vi "tm_readmetadata.vi"(5 "Index":i32, 7 "Type":i32(ring) items=["FILE"=0, "FRAME"=2], 8 "error in (no error)":errorcluster, 11 "File Handle":u32) -> (0 "error out":errorcluster, 2 "Metadata":string, 3 "File Handle":u32)   [LabVIEW 2011]
uses:
  tmcamcon.dll
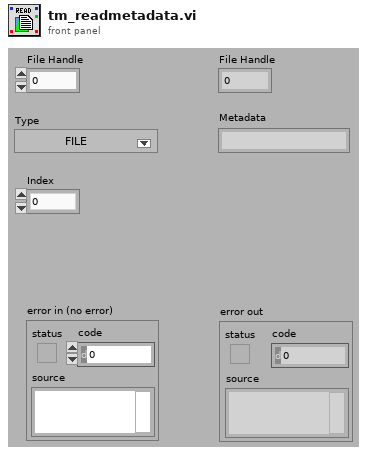
[diagram p1: front panel]
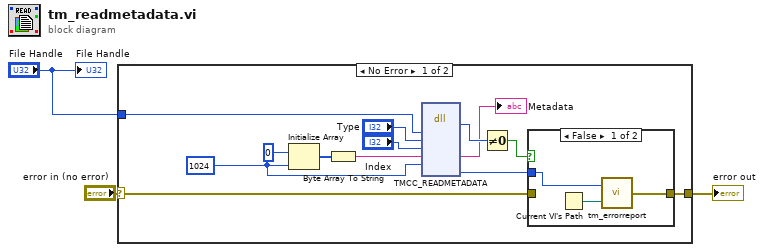
[diagram p0: block diagram]
diagram:
  n1 = case shown="No Error" "error in (no error)" {
    selector: "error in (no error)" -> [w14 w21]
    tunnel: [w11 w21] -> w2
    tunnel: "File Handle" -> [w15 _]
    frame No Error {
      w4 = 1024
      n2 = Initialize Array(u8 0, w4) -> (w8:u8[])
      n3 = Byte Array To String(unsigned byte array=w8) -> (string=w7:string)
      n4 = dll-call lib="tmcamcon.dll" fn="TMCC_READMETADATA"("handle"=w15, "type"="Type", "frame"="Index", "Metadata"=w7, "length"=w4) -> ("return type"=w16:u32, "Metadata"=→"Metadata":string, "Erval"=w13:i32)  [unwired: 8 in, 2 out]
      n5 = Not Equal To 0?(x=w16) -> (x != 0?=w12:bool)
      n6 = case shown="False" w12 {
        tunnel: w14 -> [_ w20]
        tunnel: [w18 w20] -> w11
        tunnel: w13 -> [w17 _]
        frame False {
          n7 = Current VI's Path() -> (path=w19:path)
          n8 = call <userlib>:"tm_errorreport.vi"("Source"=w19, "Error"=w17) -> ("error out"=w18:errorcluster)
        }
        frame True {
        }
      }
    }
    frame Error {
    }
  }
  "error out" <- w2
  "File Handle" <- "File Handle"
